vi "Variant to Font Data.vi"(8 "Error In":errorcluster, 10 "Font Key Name":string, 11 "Fonts LUT in":variant) -> (0 "Error Out":errorcluster, 1 "Font Found?":bool, 2 "Font out":T1, 3 "Fonts LUT out":variant)   [LabVIEW 2016, in "FontUIP.lvclass"]
uses:
  FontUIP.lvclass
  <vilib>/Utility/miscctls.llb/LVFontTypeDef.ctl
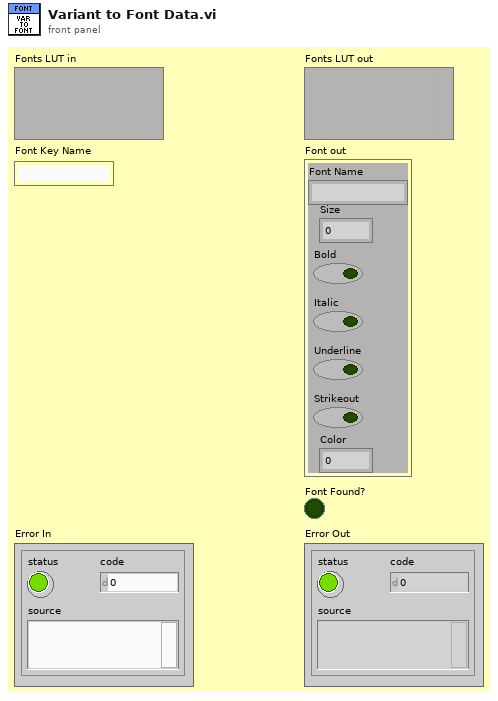
[diagram p1: front panel]
types:
  T1 = typedef "LVFontTypeDef.ctl" = cluster{"Font Name":string, "Size":u16, "Bold":bool, "Italic":bool, "Underline":bool, "Strikeout":bool, "Color":u32}
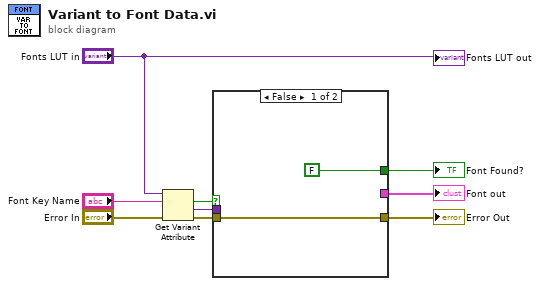
[diagram p0: block diagram]
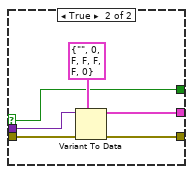
[diagram p2: hidden frame]
diagram:
  n1 = Get Variant Attribute(Variant="Fonts LUT in", name="Font Key Name", error in="Error In") -> (found=w3:bool, value=w5:variant, error out=w4:errorcluster)  [unwired: 1 in, 1 out]
  n2 = case shown="False" w3 {
    selector: w3 -> [_ w12]
    tunnel: [_ w16] -> w9
    tunnel: [w11 w15] -> w8
    tunnel: w5 -> [_ w14]
    tunnel: w4 -> [w11 w13]
    tunnel: [FALSE w12] -> w2
    frame False {
    }
    frame True {
      n3 = Variant To Data(error in=w13, type=T1 {"Font Name"="", "Size"=0, "Bold"=FALSE, "Italic"=FALSE, "Underline"=FALSE, "Strikeout"=FALSE, "Color"=0} ("Font"), Variant=w14) -> (data=w16:T1, error out=w15:errorcluster)
    }
  }
  "Font out" <- w9
  "Error Out" <- w8
  "Font Found?" <- w2
  "Fonts LUT out" <- "Fonts LUT in"
